vi "Single Channel Log String.vi"(3 "Single Channel Params":T1 {"Train Length" min=20 max=500 step=5}) -> (1 "Log String":string)   [LabVIEW 2019]
uses:
  Controls/Type Defs/Single Channel Params.ctl
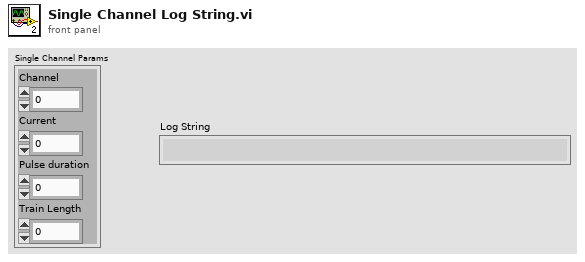
[diagram p1: front panel]
types:
  T1 = typedef "Single Channel Params.ctl" = cluster{"Channel":i32, "Current":u8, "Pulse duration":u16, "Train Length":i64}
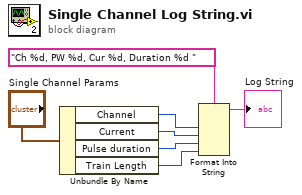
[diagram p0: block diagram]
diagram:
  n1 = Unbundle By Name("Single Channel Params") -> ("Channel"=w7:i32, "Current"=w3:u8, "Pulse duration"=w2:u16, "Train Length"=w1:i64)
  n2 = Format Into String(format string="Ch %d, PW %d, Cur %d, Duration %d ", w7, w3, w2, w1) -> (resulting string=→"Log String":string)  [unwired: 2 in, 1 out]
